vi "Play.vi"(8 "error in (no error)":errorcluster, 10 "Sound":refnum<class "Sound.lvclass">, 11 "Sound Player":refnum<class "Sound Player.lvclass">) -> (0 "error out":errorcluster, 3 "Sound Player out":refnum<class "Sound Player.lvclass">)   [LabVIEW 2017, in "Sound Player.lvclass"]
doc: "Play the given sound on the sound player."
uses:
  Sound Player.lvclass
  Sound/Sound.lvclass
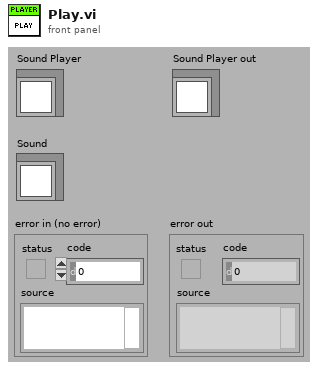
[diagram p1: front panel]
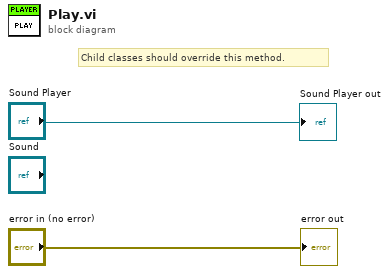
[diagram p0: block diagram]
diagram:
  # "Child classes should override this method."
  "error out" <- "error in (no error)"
  "Sound Player out" <- "Sound Player"
